vi "Read maxElapsedTime.vi"(8 "error in":errorcluster, 11 "Switch in":refnum<class "Switch.lvclass">) -> (0 "error out":errorcluster, 2 "maxElapsedTime":cluster{"true":sgl, "false":sgl}, 3 "Switch out":refnum<class "Switch.lvclass">)   [LabVIEW 2019, in "Switch.lvclass"]
doc: "Populate the max elapsed time of the switch for both the on and off positions."
uses:
  Switch.lvclass
  Switch.lvclass/Switch.ctl
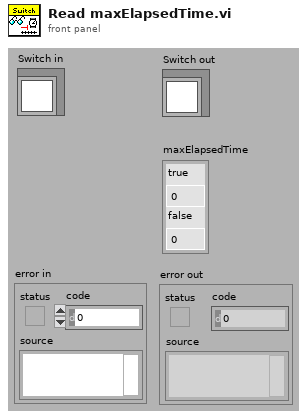
[diagram p1: front panel]
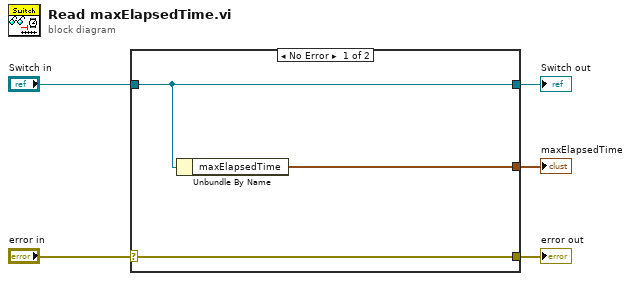
[diagram p0: block diagram]
diagram:
  n1 = case shown="No Error" "error in" {
    selector: "error in" -> [w6 w9]
    tunnel: [w6 w9] -> w4
    tunnel: [w8 w10] -> w2
    tunnel: "Switch in" -> [w8 w10]
    tunnel: [w7 _] -> w1
    frame No Error {
      n2 = Unbundle By Name(w8) -> ("maxElapsedTime"=w7:cluster{"true":sgl, "false":sgl})
    }
    frame Error {
    }
  }
  "error out" <- w4
  "Switch out" <- w2
  "maxElapsedTime" <- w1
